vi "ClimbLogic.vi"() -> ()   [LabVIEW 2018]
uses:
  <vilib>/Rock Robotics/WPI/ThirdParty/Phoenix-LabVIEW/Motor Controller/Controls/CTRE_Phoenix_MotorControl_ControlMode.ctl
  <vilib>/Rock Robotics/WPI/Relay/WPI_RelayValue.ctl
  <vilib>/Rock Robotics/WPI/Utilities/WPI_GetSetVariantRefNum.vi
  Globals.vi
  <vilib>/Rock Robotics/WPI/ThirdParty/Phoenix-LabVIEW/Motor Controller/Get/CTRE_Phoenix_MotorController_GetLimitSwitchStates.vi
panel:
  in  "ClimbLevel":enum16{"2", "3"}(ring)
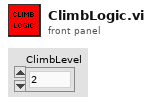
[diagram p1: front panel]
types:
  T1 = typedef "WPI_AnalogChannelDevRef.ctl" = cluster{"DevStatus":errorcluster, "Analog Channel":T2}
  T2 = typedef "FPGA_AIChannel.ctl" = enum8{"AI 0", "AI 1", "AI 2", "AI 3", "AI MXP 0", "AI MXP 1", "AI MXP 2", "AI MXP 3", "Invalid"}
  T3 = typedef "WPI_RelayDevRef.ctl" = cluster{"DevStatus":errorcluster, "Relay Channel":T4, "Relay Direction":T5}
  T4 = typedef "FPGA_DIORelayChannel.ctl" = enum8{"Relay 0", "Relay 1", "Relay 2", "Relay 3", "Invalid"}
  T5 = typedef "WPI_RelayDirection.ctl" = enum16{"Both directions", "Forward only", "Reverse only"}
  T6 = typedef "WPI_JoystickDevRef.ctl" = cluster{"Device":T7}
  T7 = typedef "WPI_JoystickDeviceEnum.ctl" = enum16{"USB 0", "USB 1", "USB 2", "USB 3", "USB 4", "USB 5"}
  T8 = typedef "WPI_MotorControlDeviceRef.ctl" = cluster{"DeviceStatus":errorcluster, "Type":T9, "PWM":cluster{"PWM Channel":T10, "DeadBand":T11}, "CAN":cluster{"Device Number":u8, "SetOutput VI Ref":variant, "GetOutput VI Ref":variant, "Enable VI Ref":variant, "Disable VI Ref":variant, "Data":variant}, "Invert":bool, "DIO PWM":cluster{"PWM \"Enable\" Channel":T10, "DIOChannel":T12, "PWM Rate":dbl}}
  T9 = typedef "WPI_MotorControlType.ctl" = enum16{"PWM", "CAN", "DIO PWM"}
  T10 = typedef "FPGA_DIOPWMChannel.ctl" = enum8{"PWM 0", "PWM 1", "PWM 2", "PWM 3", "PWM 4", "PWM 5", "PWM 6", "PWM 7", "PWM 8", "PWM 9", "PWM MXP 0", "PWM MXP 1", "PWM MXP 2", "PWM MXP 3", "PWM MXP 4", "PWM MXP 5", "PWM MXP 6", "PWM MXP 7", "PWM MXP 8", "PWM MXP 9", "Invalid"}
  T11 = typedef "WPI_PWMDeadband.ctl" = cluster{"Name":string, "maxPositivePwm":i32, "minPositivePwm":i32, "centerPwm":i32, "maxNegativePwm":i32, "minNegativePwm":i32, "angularRange":u16}
  T12 = typedef "FPGA_DIOChannel.ctl" = enum8{"DIO 0", "DIO 1", "DIO 2", "DIO 3", "DIO 4", "DIO 5", "DIO 6", "DIO 7", "DIO 8", "DIO 9", "DIO MXP 0", "DIO MXP 1", "DIO MXP 2", "DIO MXP 3", "DIO MXP 4", "DIO MXP 5", "DIO MXP 6", "DIO MXP 7", "DIO MXP 8", "DIO MXP 9", "DIO MXP 10", "DIO MXP 11", "DIO MXP 12", "DIO MXP 13", "DIO MXP 14", "DIO MXP 15", "SPI Port CS1", "SPI Port CS2", "SPI Port CS3", "SPI Port MISO", "SPI Port MOSI", "Invalid"}
  T13 = typedef "WPI_EncoderDevRef.ctl" = cluster{"DevStatus":errorcluster, "EncoderIndex":T14, "CounterIndex":T15, "DistancePerCount":dbl, "Decoding Type":T16}
  T14 = typedef "FPGA_EncoderIdx.ctl" = enum8{"Enc 0", "Enc 1", "Enc 2", "Enc 3", "Enc 4", "Enc 5", "Enc 6", "Enc 7", "Invalid"}
  T15 = typedef "FPGA_CounterCtrSystemIndex.ctl" = enum8{"Ctr 0", "Ctr 1", "Ctr 2", "Ctr 3", "Ctr 4", "Ctr 5", "Ctr 6", "Ctr 7", "Invalid"}
  T16 = typedef "WPI_EncoderType.ctl" = enum16{"1x", "2x", "4x"}
  T17 = typedef "WPI_RelayValue.ctl" = enum16{"Off", "On", "Forward", "Reverse"}
  T18 = enum16{"initial climb", "elevated drive", "retract 1", "on platform drive", "retract 2", "finish"}
  T19 = typedef "CTRE_Phoenix_MotorControl_ControlMode.ctl" = u16
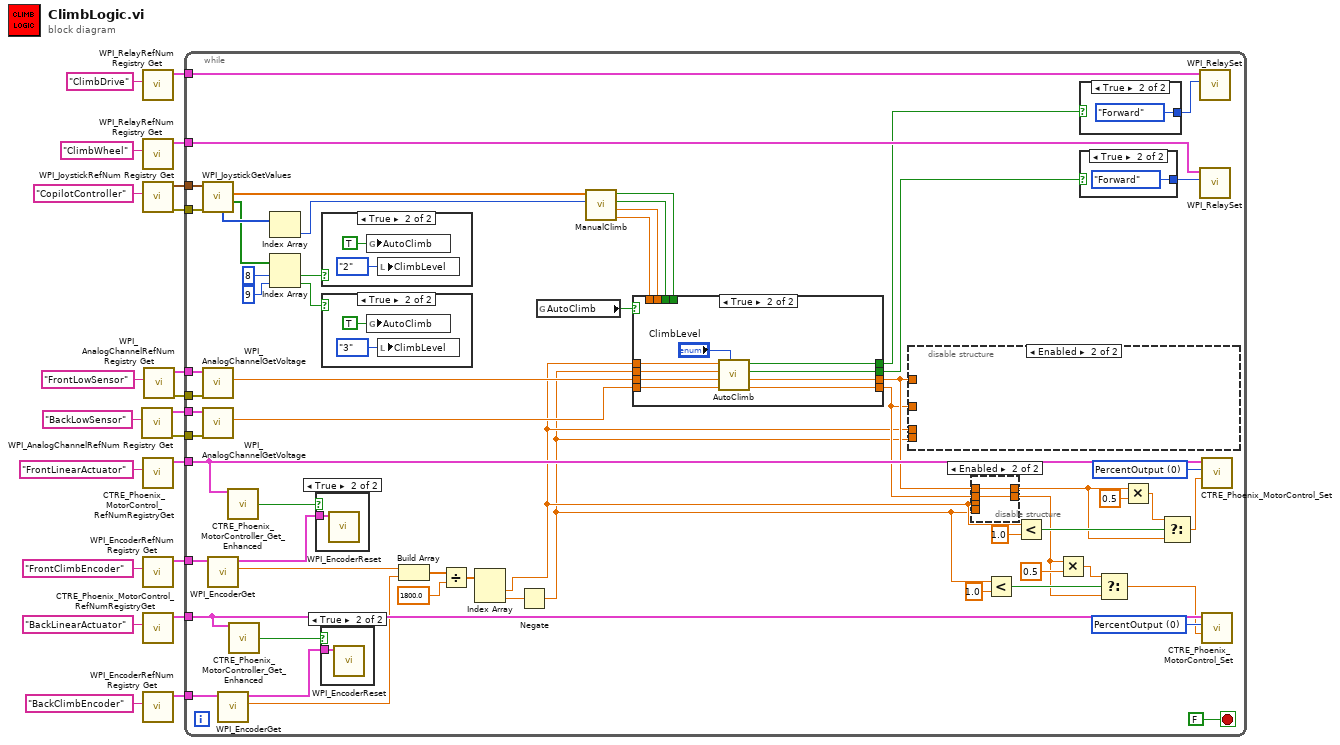
[diagram p0: block diagram]
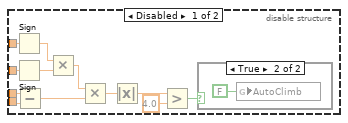
[diagram p2: hidden frame]
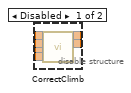
[diagram p4: hidden frame]
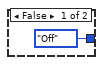
[diagram p7: hidden frame]
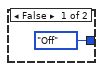
[diagram p10: hidden frame]
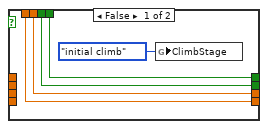
[diagram p11: hidden frame]
diagram:
  n1 = call <vilib>:"WPI_AnalogChannelRefNum Registry Get.vi"("refnum name"="BackLowSensor") -> ("error out"=w1:errorcluster, "AIDeviceRef"=w9:T1)  [unwired: 9 in]
  n2 = call <vilib>:"WPI_RelayRefNum Registry Get.vi"("refnum name"="ClimbDrive") -> ("RelayDevRef"=w11:T3)  [unwired: 9 in, 1 out]
  n3 = call <vilib>:"WPI_RelayRefNum Registry Get.vi"("refnum name"="ClimbWheel") -> ("RelayDevRef"=w8:T3)  [unwired: 9 in, 1 out]
  n4 = call <vilib>:"WPI_JoystickRefNum Registry Get.vi"("refnum name"="CopilotController") -> ("error out"=w3:errorcluster, "JoystickDevRef"=w12:T6)  [unwired: 1 in, 8 out]
  n5 = call <vilib>:"CTRE_Phoenix_MotorControl_RefNumRegistryGet.vi"("refnum name"="FrontLinearActuator") -> ("PhoenixMotorControlDevRef"=w7:T8)  [unwired: 9 in, 1 out]
  n6 = call <vilib>:"WPI_EncoderRefNum Registry Get.vi"("refnum name"="FrontClimbEncoder") -> ("EncoderDevRef"=w6:T13)  [unwired: 9 in, 1 out]
  n7 = call <vilib>:"CTRE_Phoenix_MotorControl_RefNumRegistryGet.vi"("refnum name"="BackLinearActuator") -> ("PhoenixMotorControlDevRef"=w5:T8)  [unwired: 9 in, 1 out]
  n8 = call <vilib>:"WPI_EncoderRefNum Registry Get.vi"("refnum name"="BackClimbEncoder") -> ("EncoderDevRef"=w4:T13)  [unwired: 9 in, 1 out]
  n9 = call <vilib>:"WPI_AnalogChannelRefNum Registry Get.vi"("refnum name"="FrontLowSensor") -> ("error out"=w2:errorcluster, "AIDeviceRef"=w10:T1)  [unwired: 9 in]
  n10 = while {
    tunnel: w12 -> [w74]
    tunnel: w11 -> [w26]
    tunnel: w10 -> [w73]
    tunnel: w9 -> [w72]
    tunnel: w8 -> [w71]
    tunnel: w7 -> [w70]
    tunnel: w6 -> [w69]
    tunnel: w5 -> [w68]
    tunnel: w4 -> [w67]
    tunnel: w3 -> [w66]
    tunnel: w2 -> [w46]
    tunnel: w1 -> [w45]
    stop <- FALSE stop-if-true
    w55 = T19 0 items=["PercentOutput"=0, "Position"=1, "Velocity"=2, "Current"=3, "Follower"=5, "MotionProfile"=6, "MotionMagic"=7, "MotionProfileArc"=10, "Disabled"=15] ("Control Mode")
    w56 = T19 0 items=["PercentOutput"=0, "Position"=1, "Velocity"=2, "Current"=3, "Follower"=5, "MotionProfile"=6, "MotionMagic"=7, "MotionProfileArc"=10, "Disabled"=15] ("Control Mode")
    n11 = call <vilib>:"WPI_JoystickGetValues.vi"("error in (no error)"=w66, "JoystickDevRef"=w74) -> ("Buttons"=w63:bool[], "Axes"=w81:dbl[], "POVs"=w65:i16[])  [unwired: 5 in, 2 out]
    n12 = call <vilib>:"WPI_AnalogChannelGetVoltage.vi"("error in (no error)"=w46, "AIDeviceRef"=w73) -> ("Voltage"=w79:dbl)  [unwired: 7 in, 2 out]
    n13 = call <vilib>:"WPI_AnalogChannelGetVoltage.vi"("error in (no error)"=w45, "AIDeviceRef"=w72) -> ("Voltage"=w80:dbl)  [unwired: 7 in, 2 out]
    n14 = call <vilib>:"WPI_EncoderGet.vi"("EncoderDevRef"=w69) -> ("Distance"=w52:dbl, "EncoderDevRef"=w76:T13)  [unwired: 5 in, 4 out]
    n15 = call <vilib>:"WPI_EncoderGet.vi"("EncoderDevRef"=w67) -> ("Distance"=w53:dbl, "EncoderDevRef"=w77:T13)  [unwired: 5 in, 4 out]
    n16 = call-poly <vilib>:"CTRE_Phoenix_MotorController_Get_Enhanced.vi"("PhoenixMotorControlDevRef"=w70) -> ("Reverse Limit Closed?"=w58:bool)  [unwired: 11 in, 3 out]
    n17 = call-poly <vilib>:"CTRE_Phoenix_MotorController_Get_Enhanced.vi"("PhoenixMotorControlDevRef"=w68) -> ("Reverse Limit Closed?"=w57:bool)  [unwired: 11 in, 3 out]
    n18 = Index Array(array=w65) -> (element=w64:i16)  [unwired: 1 in]
    n19 = Index Array(array=w63, index #1=8 ("index"), index #2=9 ("index")) -> (element #1=w62:bool, element #2=w60:bool)
    n20 = case shown="True" w58 {
      tunnel: w76 -> [_ w110]
      frame False {
      }
      frame True {
        n21 = call <vilib>:"WPI_EncoderReset.vi"("EncoderDevRef"=w110) -> ()  [unwired: 9 in, 2 out]
      }
    }
    n22 = case shown="True" w57 {
      tunnel: w77 -> [_ w109]
      frame False {
      }
      frame True {
        n23 = call <vilib>:"WPI_EncoderReset.vi"("EncoderDevRef"=w109) -> ()  [unwired: 9 in, 2 out]
      }
    }
    n24 = case shown="True" w62 {
      frame False {
      }
      frame True {
        n25 = global write "Globals.vi" "AutoClimb"(TRUE ("AutoClimb")) -> ()
        n26 = local write "ClimbLevel"(enum16{"2", "3"}."2" ("ClimbLevel")) -> ()
      }
    }
    n27 = case shown="True" w60 {
      frame False {
      }
      frame True {
        n28 = global write "Globals.vi" "AutoClimb"(TRUE ("AutoClimb")) -> ()
        n29 = local write "ClimbLevel"(enum16{"2", "3"}."3" ("ClimbLevel")) -> ()
      }
    }
    n30 = Build Array(w52, w53) -> (w41:dbl[])
    n31 = Divide(x=w41, y=1800.0) -> (x/y=w54:dbl[])
    n32 = Index Array(array=w54) -> (element #1=w23:dbl, element #2=w24:dbl)  [unwired: 2 in]
    n33 = Negate(x=w24) -> (-x=w22:dbl)
    n34 = global read "Globals.vi" "AutoClimb"() -> (w44:bool)
    n35 = call "ManualClimb.vi"("CopilotPOV"=w64, "CopilotAxes"=w81) -> ("ActuateBackClimb"=w49:dbl, "ActuateFrontClimb"=w43:dbl, "DropWheel"=w50:bool, "ClimbDrive"=w51:bool)  [unwired: 6 in]
    n36 = case shown="True" w44 {
      tunnel: w23 -> [_ w126]
      tunnel: w22 -> [_ w123]
      tunnel: w79 -> [_ w125]
      tunnel: w80 -> [_ w124]
      tunnel: [w117 w121] -> w48
      tunnel: w51 -> [w117 _]
      tunnel: [w116 w120] -> w42
      tunnel: w50 -> [w116 _]
      tunnel: [w115 w118] -> w27
      tunnel: w43 -> [w115 _]
      tunnel: [w114 w119] -> w25
      tunnel: w49 -> [w114 _]
      frame False {
        n37 = global write "Globals.vi" "ClimbStage"(T18."initial climb" ("ClimbStage")) -> ()
      }
      frame True {
        n38 = call "AutoClimb.vi"("ClimbLevel"="ClimbLevel", "BackLowSensor"=w124, "FrontLowSensor"=w125, "BackClimbEncoder"=w123, "FrontClimbEncoder"=w126) -> ("ActuateBackClimb"=w119:dbl, "ActuateFrontClimb"=w118:dbl, "DropWheel"=w120:bool, "ClimbDrive"=w121:bool)  [unwired: 3 in]
      }
    }
    n39 = disable-structure shown="Enabled" {
      disable-tunnel: w27 -> [w85 _]
      disable-tunnel: w25 -> [w84 _]
      disable-tunnel: w23 -> [w83 _]
      disable-tunnel: w22 -> [w82 _]
      frame Disabled {
        n40 = Sign(1:w85) -> (0:w87:dbl)
        n41 = Sign(1:w84) -> (0:w86:dbl)
        n42 = Subtract(x=w83, y=w82) -> (x-y=w93:dbl)
        n43 = Multiply(x=w87, y=w86) -> (x*y=w88:dbl)
        n44 = Multiply(x=w88, y=w93) -> (x*y=w89:dbl)
        n45 = Absolute Value(x=w89) -> (abs(x)=w90:dbl)
        n46 = Greater?(x=w90, y=4.0) -> (0:w91:bool)
        n47 = case shown="True" w91 {
          frame False {
          }
          frame True {
            n48 = global write "Globals.vi" "AutoClimb"(FALSE ("AutoClimb")) -> ()
          }
        }
      }
      frame Enabled {
      }
    }
    n49 = disable-structure shown="Enabled" {
      disable-tunnel: [w100 w101] -> w29
      disable-tunnel: [w99 w102] -> w28
      disable-tunnel: w27 -> [w98 w102]
      disable-tunnel: w25 -> [w97 w101]
      disable-tunnel: w23 -> [w96 _]
      disable-tunnel: w22 -> [w95 _]
      frame Disabled {
        n50 = call "CorrectClimb.vi"("BackEncoder"=w95, "FrontEncoder"=w96, "BackControl"=w97, "FrontControl"=w98) -> ("BackOutput"=w100:dbl, "FrontOutput"=w99:dbl)  [unwired: 6 in]
      }
      frame Enabled {
      }
    }
    n51 = Less?(x=w22, y=1.0) -> (x < y?=w38:bool)
    n52 = Less?(x=w23, y=1.0) -> (x < y?=w34:bool)
    n53 = Multiply(x=w29, y=0.5) -> (x*y=w30:dbl)
    n54 = case shown="True" w48 {
      tunnel: [WPI_RelayValue."Off" ("RelayValue") WPI_RelayValue."Forward" ("RelayValue")] -> w75
      frame False {
      }
      frame True {
      }
    }
    n55 = case shown="True" w42 {
      tunnel: [WPI_RelayValue."Off" ("RelayValue") WPI_RelayValue."Forward" ("RelayValue")] -> w78
      frame False {
      }
      frame True {
      }
    }
    n56 = Select(t=w30, s=w38, f=w29) -> (s? t:f=w37:dbl)
    n57 = Multiply(x=w28, y=0.5) -> (x*y=w31:dbl)
    n58 = Select(t=w31, s=w34, f=w28) -> (s? t:f=w32:dbl)
    n59 = call <vilib>:"WPI_RelaySet.vi"("RelayValue"=w75, "RelayDevRef"=w26) -> ()  [unwired: 8 in, 2 out]
    n60 = call <vilib>:"WPI_RelaySet.vi"("RelayValue"=w78, "RelayDevRef"=w71) -> ()  [unwired: 8 in, 2 out]
    n61 = call <vilib>:"CTRE_Phoenix_MotorControl_Set.vi"("Output"=w32, "Control Mode"=w56, "PhoenixMotorControlDevRef"=w70) -> ()  [unwired: 7 in, 2 out]
    n62 = call <vilib>:"CTRE_Phoenix_MotorControl_Set.vi"("Output"=w37, "Control Mode"=w55, "PhoenixMotorControlDevRef"=w68) -> ()  [unwired: 7 in, 2 out]
  }
